vi "TIO Stream Read Non-blocking.vi"(8 "error in (no error)":errorcluster, 11 "TS Connection":T1={"Type"=enum."TCP", "Serial"="serial:///dev/cu.usbserial-00000", "TCP"=refnum, "Timeout"=500}) -> (0 "error out":errorcluster, 1 "Payload":string, 2 "Type":u16(ring)=2 items=["Invalid", "Log", "RPC Request", "RPC Reply", "RPC Error", "Stream Description", "User"], 3 "TS Connection":T1={"Type"=enum."TCP", "Serial"="serial:///dev/cu.usbserial-00000", "TCP"=refnum, "Timeout"=500})   [LabVIEW 2016]
panel:
  out "Routing Size":u8
  out "Payload Length":u16
  # "TODO Handle routing"
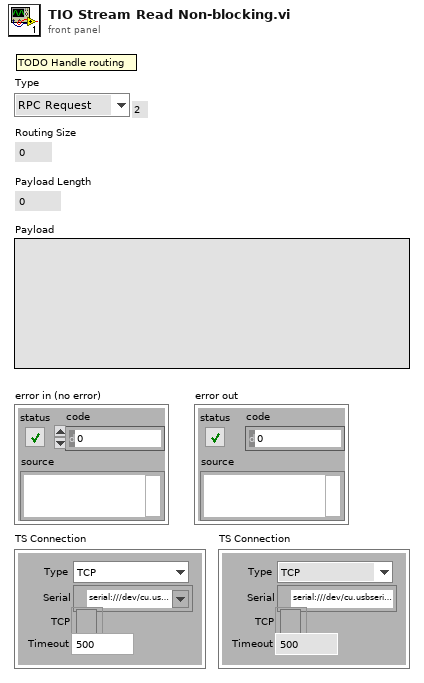
[diagram p1: front panel]
types:
  T1 = cluster{"Type":enum16{"TCP", "Serial"}, "Serial":refnum<visa-resource-name>, "TCP":refnum<k5>, "Timeout":u32}
  T2 = enum16{"Standard", "Buffered", "CRLF", "Immediate"}
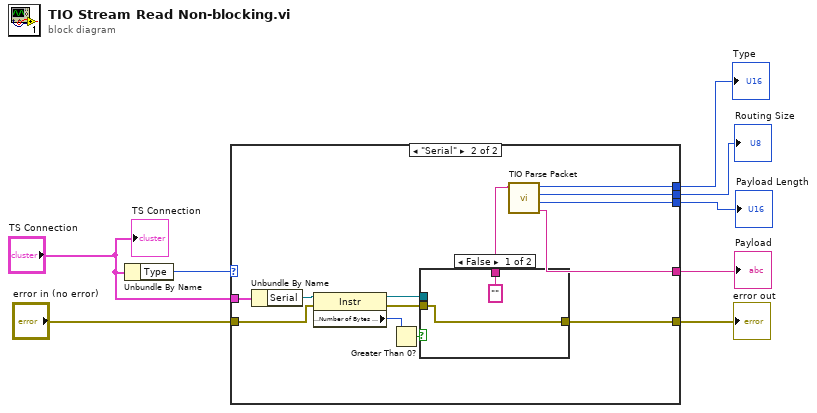
[diagram p0: block diagram]
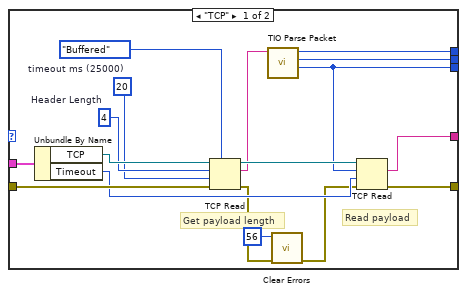
[diagram p2: hidden frame]
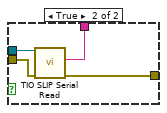
[diagram p3: hidden frame]
diagram:
  n1 = Unbundle By Name("TS Connection") -> ("Type"=w6:enum16{"TCP", "Serial"})
  n2 = case shown="\"Serial\"" w6 {
    tunnel: "error in (no error)" -> [w22 w29]
    tunnel: [w21 w38] -> w8
    tunnel: "TS Connection" -> [w25 w37]
    tunnel: [w20 w33] -> w1
    tunnel: [w14 w34] -> w4
    tunnel: [w16 w35] -> w3
    tunnel: [w15 w36] -> w2
    frame "TCP" {
      w13 = 20  # timeout ms (25000)
      w18 = u32 4  # Header Length
      # "Read payload"
      # "Get payload length"
      n3 = Unbundle By Name(w25) -> ("TCP"=w24:refnum<k5>, "Timeout"=w19:u32)
      n4 = TCP Read(connection ID=w24, bytes to read=w18, error in (no error)=w22, 7:T2."Buffered" ("mode (standard)"), 9:w13) -> (connection ID out=w23:refnum<k5>, data out=w17:string, error out=w11:errorcluster)
      n5 = call "TIO Parse Packet.vi"("Packet"=w17) -> ("Payload Length"=w14:u16, "Routing Size"=w16:u8, "Type"=w15:u16)  [unwired: 7 in, 1 out]
      n6 = call <vilib>:"Clear Errors.vi"("error in (no error)"=w11, "specific error code to clear (0: all)"=56) -> ("error out"=w10:errorcluster)  [unwired: 4 in, 1 out]
      n7 = TCP Read(connection ID=w23, bytes to read=w14, error in (no error)=w10, 9:w19) -> (data out=w20:string, error out=w21:errorcluster)  [unwired: 1 in, 1 out]
    }
    frame "Serial" {
      n8 = Unbundle By Name(w37) -> ("Serial"=w31:refnum<visa-resource-name>)
      n9 = property class="Instr"(reference=w31, error in=w29) -> (reference out=w30:refnum<visa-resource-name>, error out=w28:errorcluster, "Serial Settings:Number of Bytes at Serial Port"=w27:u32)
      n10 = Greater Than 0?(x=w27) -> (x > 0?=w26:bool)
      n11 = case shown="False" w26 {
        tunnel: [w40 w44] -> w38
        tunnel: ["" ("Payload") w43] -> w32
        tunnel: w30 -> [_ w42]
        tunnel: w28 -> [w40 w41]
        frame False {
        }
        frame True {
          n12 = call "TIO SLIP Serial Read.vi"("error in (no error)"=w41, "VISA resource name"=w42) -> ("error out"=w44:errorcluster, "Payload"=w43:string)  [unwired: 7 in, 1 out]
        }
      }
      n13 = call "TIO Parse Packet.vi"("Packet"=w32) -> ("Payload"=w33:string, "Payload Length"=w34:u16, "Routing Size"=w35:u8, "Type"=w36:u16)  [unwired: 7 in]
    }
  }
  "error out" <- w8
  "Payload" <- w1
  "Type" <- w2
  "Routing Size" <- w3
  "Payload Length" <- w4
  "TS Connection" <- "TS Connection"
